vi "open_camera.vi"() -> (0 "error":errorcluster, 1 "AOI Height":i64, 2 "AOI Width":i64, 3 "Handle":i32, 5 "PreAmp Gain Control":string(combo))   [LabVIEW 2019]
panel:
  in  "Apply Settings":bool
  in  "Centre AOI":bool
  out "Ready":bool
  in  "Run":bool
  out "Pixel Encoding":string
  out "AOIStride":i64
  out "PixelData":u16[](array[numeric])
  out "ByteData":u8[](array[numeric])
  in  "ExposureTime":dbl=0.1
  out "ImageSizeBytes":i64
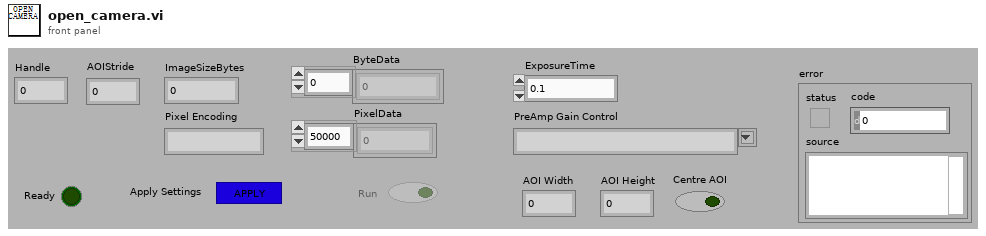
[diagram p1: front panel]
types:
  T1 = enum8{"Enabled", "Disabled", "Disabled and Grayed Out"}
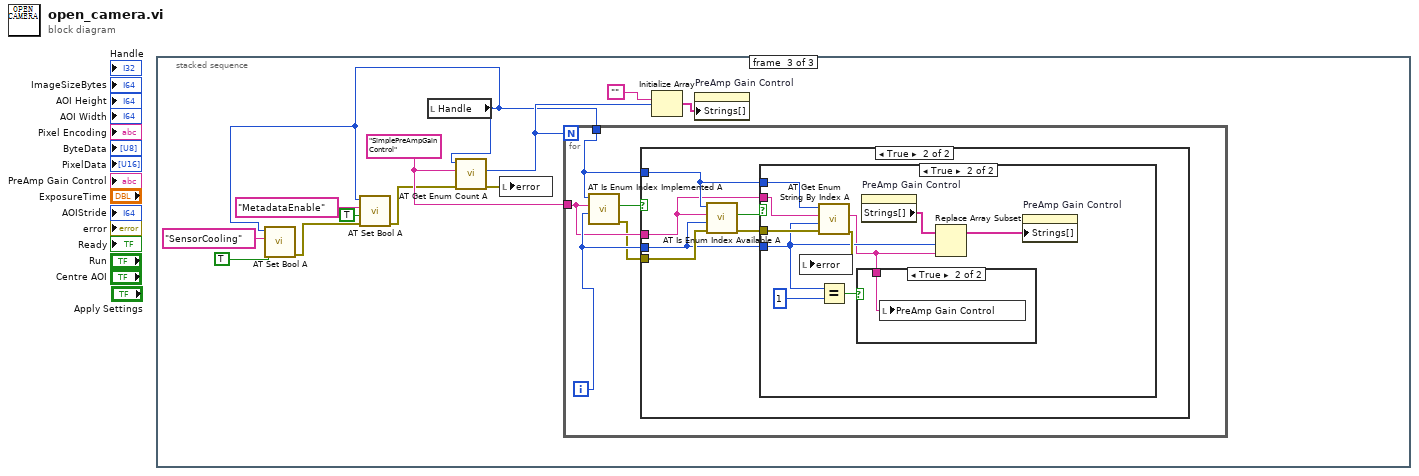
[diagram p0: block diagram]
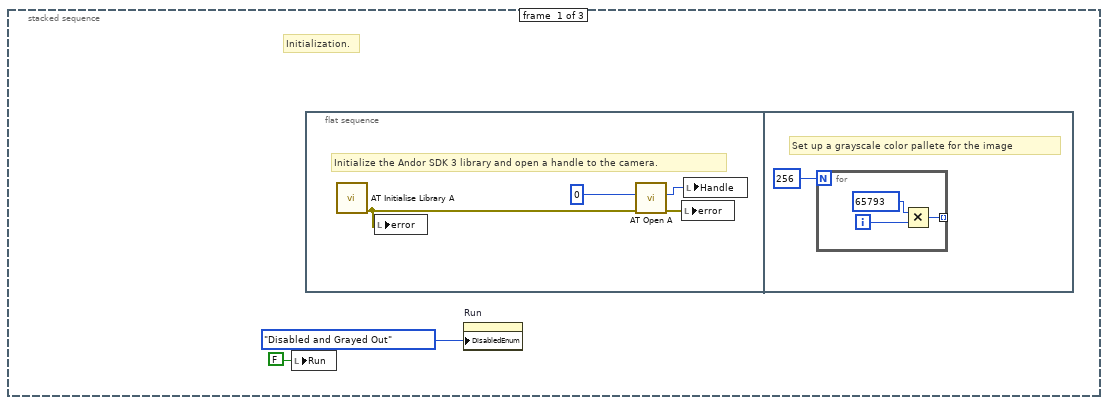
[diagram p2: hidden frame]
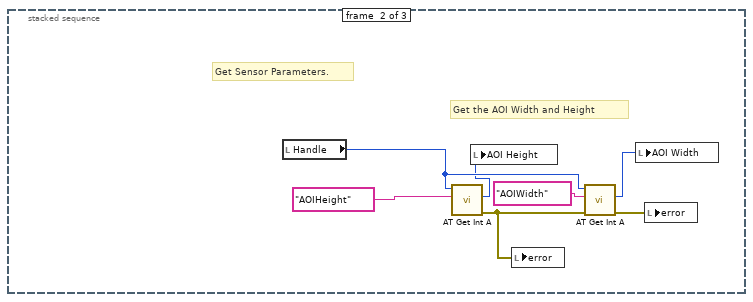
[diagram p3: hidden frame]
diagram:
  n1 = stacked-sequence {
    frame #0 {
      # "Initialization."
      n2 = local write "Run"(FALSE ("Run")) -> ()
      n3 = flat-sequence {
        frame #0 {
          # "Initialize the Andor SDK 3 library and open a handle to the camera."
          n4 = call <userlib>:"AT Initialise Library A.vi"() -> ("error out"=w4:errorcluster)  [unwired: 10 in, 1 out]
          n5 = local write "error"(w4) -> ()
          n6 = call <userlib>:"AT Open A.vi"("error in (no error)"=w4, "CameraIndex"=0) -> ("error out"=w3:errorcluster, "Handle"=w5:i32)  [unwired: 7 in, 1 out]
          n7 = local write "error"(w3) -> ()
          n8 = local write "Handle"(w5) -> ()
        }
        frame #1 {
          # "Set up a grayscale color pallete for the image"
          n9 = for {
            N: 256 -> [_]
            tunnel: [w9] -> _ mode=indexing
            i -> [w10]
            n10 = Multiply(x=65793, y=w10) -> (x*y=w9:i32)
          }
        }
      }
      n11 = property on="Run" class="Bool (strict)"("DisabledEnum"=T1."Disabled and Grayed Out" ("Disabled")) -> ()  [unwired: 2 in, 2 out]
    }
    frame #1 {
      # "Get the AOI Width and Height"
      # "Get Sensor Parameters."
      n12 = local read "Handle"() -> (w14:i32)
      n13 = call <userlib>:"AT Get Int A.vi"("Feature"="AOIHeight" ("Integer feature 2"), "Handle"=w14) -> ("error out"=w13:errorcluster, "Value"=w11:i64)  [unwired: 7 in, 1 out]
      n14 = local write "AOI Height"(w11) -> ()
      n15 = local write "error"(w13) -> ()
      n16 = call <userlib>:"AT Get Int A.vi"("error in (no error)"=w13, "Feature"="AOIWidth" ("Integer feature"), "Handle"=w14) -> ("error out"=w17:errorcluster, "Value"=w12:i64)  [unwired: 6 in, 1 out]
      n17 = local write "AOI Width"(w12) -> ()
      n18 = local write "error"(w17) -> ()
    }
    frame #2 {
      w25 = "SimplePreAmpGainControl" ("Enum feature")
      n19 = local read "Handle"() -> (w18:i32)
      n20 = call <userlib>:"AT Set Bool A.vi"("Value"=TRUE, "Feature"="SensorCooling", "Handle"=w18) -> ("error out"=w21:errorcluster)  [unwired: 7 in, 1 out]
      n21 = call <userlib>:"AT Set Bool A.vi"("error in (no error)"=w21, "Value"=TRUE, "Feature"="MetadataEnable", "Handle"=w18) -> ("error out"=w24:errorcluster)  [unwired: 6 in, 1 out]
      n22 = call <userlib>:"AT Get Enum Count A.vi"("error in (no error)"=w24, "Feature"=w25, "Handle"=w18) -> ("error out"=w29:errorcluster, "Count"=w28:i32)  [unwired: 6 in, 1 out]
      n23 = local write "error"(w29) -> ()
      n24 = for {
        N: w28 -> [_]
        tunnel: w18 -> [w31]
        tunnel: w25 -> [w32]
        i -> [w33]
        n25 = call <userlib>:"AT Is Enum Index Implemented A.vi"("Index"=w33, "Feature"=w32, "Handle"=w31) -> ("error out"=w30:errorcluster, "Implemented"=w34:bool)  [unwired: 6 in, 1 out]
        n26 = case shown="True" w34 {
          tunnel: w33 -> [_ w36]
          tunnel: w32 -> [_ w37]
          tunnel: w31 -> [_ w38]
          tunnel: w30 -> [_ w40]
          frame False {
          }
          frame True {
            n27 = call <userlib>:"AT Is Enum Index Available A.vi"("error in (no error)"=w40, "Index"=w36, "Feature"=w37, "Handle"=w38) -> ("error out"=w35:errorcluster, "Available"=w39:bool)  [unwired: 5 in, 1 out]
            n28 = case shown="True" w39 {
              tunnel: w38 -> [_ w50]
              tunnel: w37 -> [_ w49]
              tunnel: w36 -> [_ w46]
              tunnel: w35 -> [_ w48]
              frame False {
              }
              frame True {
                n29 = call <userlib>:"AT Get Enum String By Index A.vi"("error in (no error)"=w48, "Index"=w46, "Feature"=w49, "Handle"=w50) -> ("error out"=w47:errorcluster, "String"=w43:string)  [unwired: 5 in, 1 out]
                n30 = local write "error"(w47) -> ()
                n31 = Equal?(x=w46, y=1) -> (x = y?=w44:bool)
                n32 = case shown="True" w44 {
                  tunnel: w43 -> [_ w51]
                  frame False {
                  }
                  frame True {
                    n33 = local write "PreAmp Gain Control"(w51) -> ()
                  }
                }
                n34 = property on="PreAmp Gain Control" class="CmbBox"() -> ("Strings[]"=w42:string[])  [unwired: 2 in, 2 out]
                n35 = Replace Array Subset(array=w42, new element=w43, index=w46) -> (w41:string[])
                n36 = property on="PreAmp Gain Control" class="CmbBox"("Strings[]"=w41) -> ()  [unwired: 2 in, 2 out]
              }
            }
          }
        }
      }
      n37 = Initialize Array("", w28) -> (w26:string[])
      n38 = property on="PreAmp Gain Control" class="CmbBox"("Strings[]"=w26) -> ()  [unwired: 2 in, 2 out]
    }
  }
